vi "tb_interpolation_host.vi"() -> ()   [LabVIEW 2011]
uses:
  <vilib>/ptbypt/NI_PtbyPt.lvlib
  Controls/Interpolation Input Data.ctl
panel:
  out "Resampled Data":dbl[](graph)
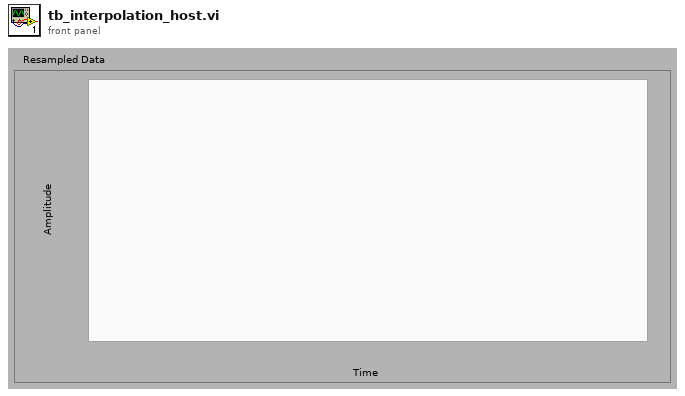
[diagram p1: front panel]
types:
  T1 = typedef "Interpolation Input Data.ctl" = fxp<+/-,18,1>
  T2 = typedef "Interpolation Output Data.ctl" = fxp<+/-,19,1>
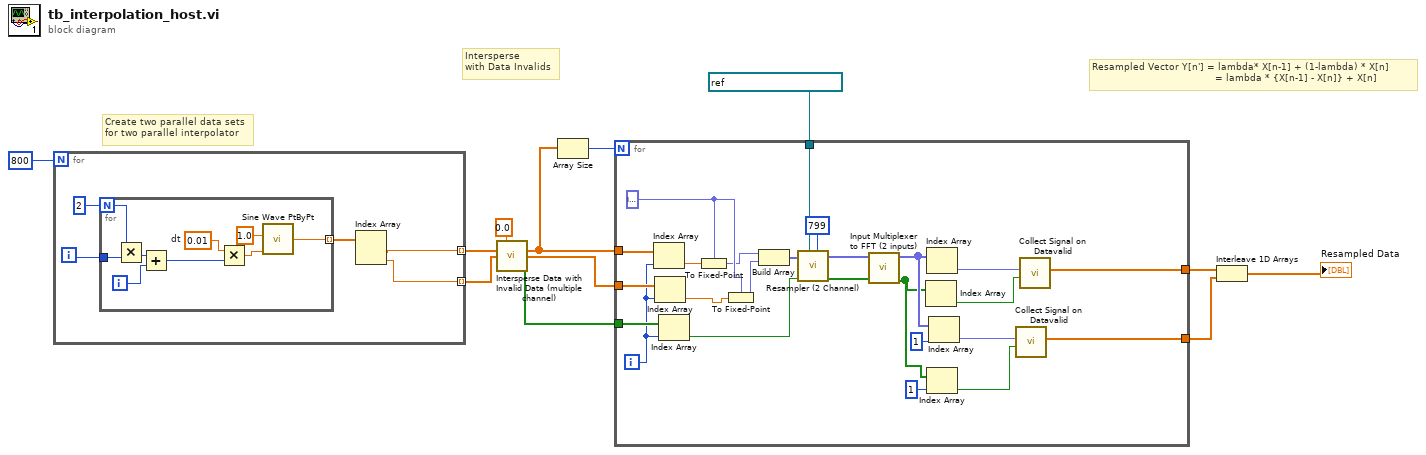
[diagram p0: block diagram]
diagram:
  # "Resampled Vector Y[n'] = lambda* X[n-1] + (1-lambda) * X[n]\n                                         = lambda * {X[n-1] - X[n]} + X[n]"
  # "Intersperse\nwith Data Invalids"
  # "Create two parallel data sets\nfor two parallel interpolator"
  n1 = for {
    N: 800 -> [_]
    tunnel: [w14] -> w10 mode=indexing
    tunnel: [w13] -> w9 mode=indexing
    i -> [w16]
    n2 = for {
      N: 2 -> [w21]
      tunnel: [w23] -> w17 mode=indexing
      tunnel: w16 -> [w22]
      i -> [w19]
      w25 = 0.01  # dt
      n3 = Multiply(x=w21, y=w22) -> (x*y=w20:i32)
      n4 = Add(x=w20, y=w19) -> (x+y=w18:i32)
      n5 = Multiply(x=w25, y=w18) -> (x*y=w24:dbl)
      n6 = call <vilib>:"Sine Wave PtByPt.vi"("time"=w24, "frequency"=1.0) -> ("sine wave"=w23:dbl)  [unwired: 2 in]
    }
    n7 = Index Array(array=w17) -> (element #1=w14:dbl, element #2=w13:dbl)  [unwired: 2 in]
  }
  n8 = call <userlib>:"Intersperse Data with Invalid Data (multiple channel).vi"("Intersperse Ratio"=0.0, "Channel0 Input"=w10, "Channel1 Input"=w9) -> ("Channel0 Output"=w4:dbl[], "Channel1 Output"=w7:dbl[], "Data Valid"=w6:bool[])  [unwired: 10 in]
  n9 = Array Size(array=w4) -> (size(s)=w5:i32)
  n10 = for {
    N: w5 -> [_]
    tunnel: refnum<k21> "ResampleVectorInfo" ("ResampleVectorInfo") -> [w51]
    tunnel: w4 -> [w49]
    tunnel: w7 -> [w48]
    tunnel: w6 -> [w47]
    tunnel: [w35] -> w3
    tunnel: [w34] -> w2
    i -> [w45]
    w42 = T1 0.0 ("Interpolate.Input Data")
    n11 = Index Array(array=w49, index=w45) -> (element=w44:dbl)
    n12 = Index Array(array=w48, index=w45) -> (element=w43:dbl)
    n13 = Index Array(array=w47, index=w45) -> (element=w46:bool)
    n14 = To Fixed-Point(fixed-point type=w42, number=w44) -> (fixed-point=w40:T1)
    n15 = To Fixed-Point(fixed-point type=w42, number=w43) -> (fixed-point=w41:T1)
    n16 = Build Array(w40, w41) -> (w39:T1[])
    n17 = call "Resampler (2 Channel).vi"("CalibrationTable Length-1"=u16 799 ("Table Length-1"), "ResampleVectorInfo"=w51, "DataValid"=w46, "Input Data"=w39) -> ("Data Valid"=w37:bool[], "Interpolated Data"=w38:T2[])  [unwired: 6 in]
    n18 = call "Input Multiplexer to FFT (2 inputs).vi"("Input Data Valid Array"=w37, "Input Data"=w38) -> ("Output Data Valid Array"=w31:bool[], "Interchanged Data"=w32:T2[])  [unwired: 8 in]
    n19 = Index Array(array=w31) -> (element=w33:bool)  [unwired: 1 in]
    n20 = Index Array(array=w32) -> (element=w36:T2)  [unwired: 1 in]
    n21 = Index Array(array=w31, index=1) -> (element=w28:bool)
    n22 = Index Array(array=w32, index=1) -> (element=w27:T2)
    n23 = call <userlib>:"Collect Signal on Datavalid.vi"("Data Valid"=w28, "Input"=w27) -> ("Output"=w34:dbl[])  [unwired: 9 in]
    n24 = call <userlib>:"Collect Signal on Datavalid.vi"("Data Valid"=w33, "Input"=w36) -> ("Output"=w35:dbl[])  [unwired: 9 in]
  }
  n25 = Interleave 1D Arrays(w3, w2) -> (→"Resampled Data":dbl[])
